vi "Show Animated Busy Icon with Message.vi"(4 "Animated Busy Icon Control Name (Animated Busy Icon)":string="Animated Busy Icon", 5 "Already active? (F)":bool, 6 "Message Control Name (Message)":string="Message", 7 "Message":string, 9 "Error In":errorcluster, 11 "Target VI Refnum":refnum<vi>) -> (1 "Error Out":errorcluster)   [LabVIEW 2021]
doc: "This VI uses error in normally (doesn't do anything if there is an error in) and passes through the error in (ignores additional unternal errors)."
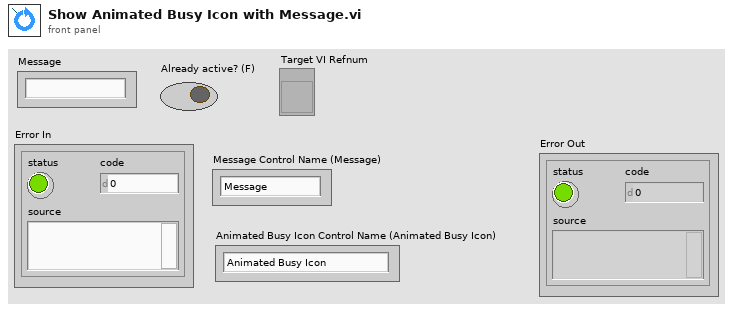
[diagram p1: front panel]
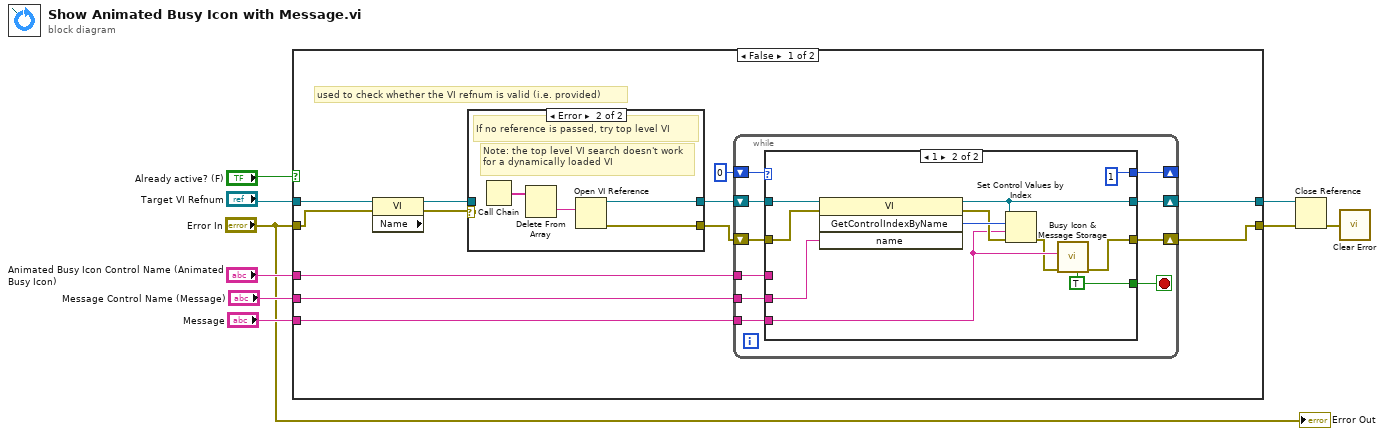
[diagram p0: block diagram]
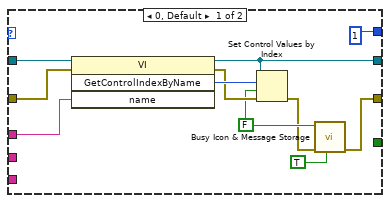
[diagram p3: hidden frame]
diagram:
  n1 = case shown="False" "Already active? (F)" {
    tunnel: [w19 w61] -> w9
    tunnel: [w18 w60] -> w8
    tunnel: "Message Control Name (Message)" -> [w16 _]
    tunnel: "Animated Busy Icon Control Name (Animated Busy Icon)" -> [w15 _]
    tunnel: "Message" -> [w14 _]
    tunnel: "Target VI Refnum" -> [w13 w61]
    tunnel: "Error In" -> [w10 w60]
    frame False {
      # "used to check whether the VI refnum is valid (i.e. provided)"
      n2 = property class="VI" props=["Name"](reference=w13, error in=w10) -> (reference out=w11:refnum<vi>, error out=w12:errorcluster)  [unwired: 1 out]
      n3 = case shown="Error" w12 {
        selector: w12 -> [w22 _]
        tunnel: [w22 w27] -> w21
        tunnel: [w23 w26] -> w20
        tunnel: w11 -> [w23 _]
        frame No Error {
        }
        frame Error {
          # "Note: the top level VI search doesn't work for a dynamically loaded VI"
          # "If no reference is passed, try top level VI"
          n4 = Call Chain() -> (call chain=w24:string[])
          n5 = Delete From Array(array=w24) -> (deleted portion=w25:string)  [unwired: 2 in, 1 out]
          n6 = Open VI Reference(vi path=w25) -> (vi reference=w26:refnum<vi>, error out=w27:errorcluster)  [unwired: 5 in]
        }
      }
      n7 = while {
        shift-right: [w34] -> w18
        shift-left: w21 -> [w37]
        shift-right: [w35] -> w19
        shift-left: w20 -> [w36]
        shift-right: [w32] -> _
        shift-left: 0 -> [w33]
        tunnel: w16 -> [w30]
        tunnel: w15 -> [w29]
        tunnel: w14 -> [w28]
        stop <- w31 stop-if-true
        n8 = case shown="1" w33 {
          tunnel: w37 -> [w46 w57]
          tunnel: w36 -> [w45 w56]
          tunnel: [w44 w55] -> w35
          tunnel: [w39 w50] -> w34
          tunnel: [1 1] -> w32
          tunnel: [_ w49] -> w31
          tunnel: w30 -> [_ w53]
          tunnel: w29 -> [w42 _]
          tunnel: w28 -> [_ w52]
          frame 0, Default {
            w41 = FALSE ("Visible")
            n9 = invoke class="VI" method="GetControlIndexByName"(reference=w45, error in=w46, "name"=w42) -> (reference out=w44:refnum<vi>, error out=w47:errorcluster, "GetControlIndexByName"=w48:i32)  [unwired: 1 in, 1 out]
            n10 = Set Control Values by Index(0:w44, 1:w48, 2:w41, 3:w47) -> (11:w40:errorcluster)
            n11 = call "Busy Icon & Message Storage.vi"("Get(F)/Set Busy Icon"=TRUE, "Error In"=w40, "Busy Icon Status (F = busy)"=w41) -> ("Error Out"=w39:errorcluster)  [unwired: 6 in, 2 out]
          }
          frame 1 {
            w49 = TRUE ("Get(F)/Set Message")
            n12 = invoke class="VI" method="GetControlIndexByName"(reference=w56, error in=w57, "name"=w53) -> (reference out=w55:refnum<vi>, error out=w58:errorcluster, "GetControlIndexByName"=w59:i32)  [unwired: 1 in, 1 out]
            n13 = Set Control Values by Index(0:w55, 1:w59, 2:w52, 3:w58) -> (11:w51:errorcluster)
            n14 = call "Busy Icon & Message Storage.vi"("Get(F)/Set Message"=w49, "Error In"=w51, "Message String"=w52) -> ("Error Out"=w50:errorcluster)  [unwired: 6 in, 2 out]
          }
        }
      }
    }
    frame True {
    }
  }
  n15 = Close Reference(reference=w9, error in (no error)=w8) -> (error out=w1:errorcluster)
  n16 = call "Clear Error.vi"("Error In"=w1) -> ()  [unwired: 8 in, 1 out]
  "Error Out" <- "Error In"
